vi "test MSS.vi"() -> ()   [LabVIEW 2023]
uses:
  Measure and Stimulus Subsystems/Measure and Stimulus Subsystems.lvclass
  Virtual Instrs/Virt Red-y Read Write/Virt Red-y Read Write.lvclass
  Configurations/Pressure Control CFG/Red-y Pressure Control CFG.lvclass
  Configurations/Pressure Control CFG Simulated/Red-y Pressure Control CFG Simulated.lvclass
panel:
  out "Pressure Scaling Max":variant
  out "Signal Type AI":variant
  out "Pressure":variant
  out "Output":variant
  out "Temperature":variant
  out "Flow":variant
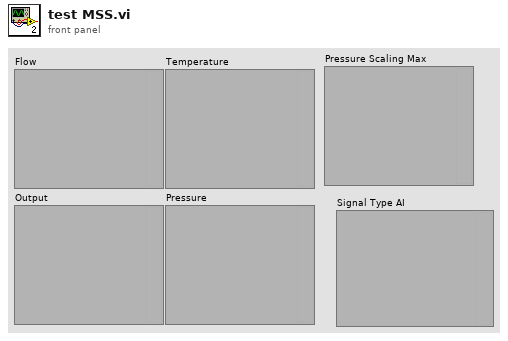
[diagram p1: front panel]
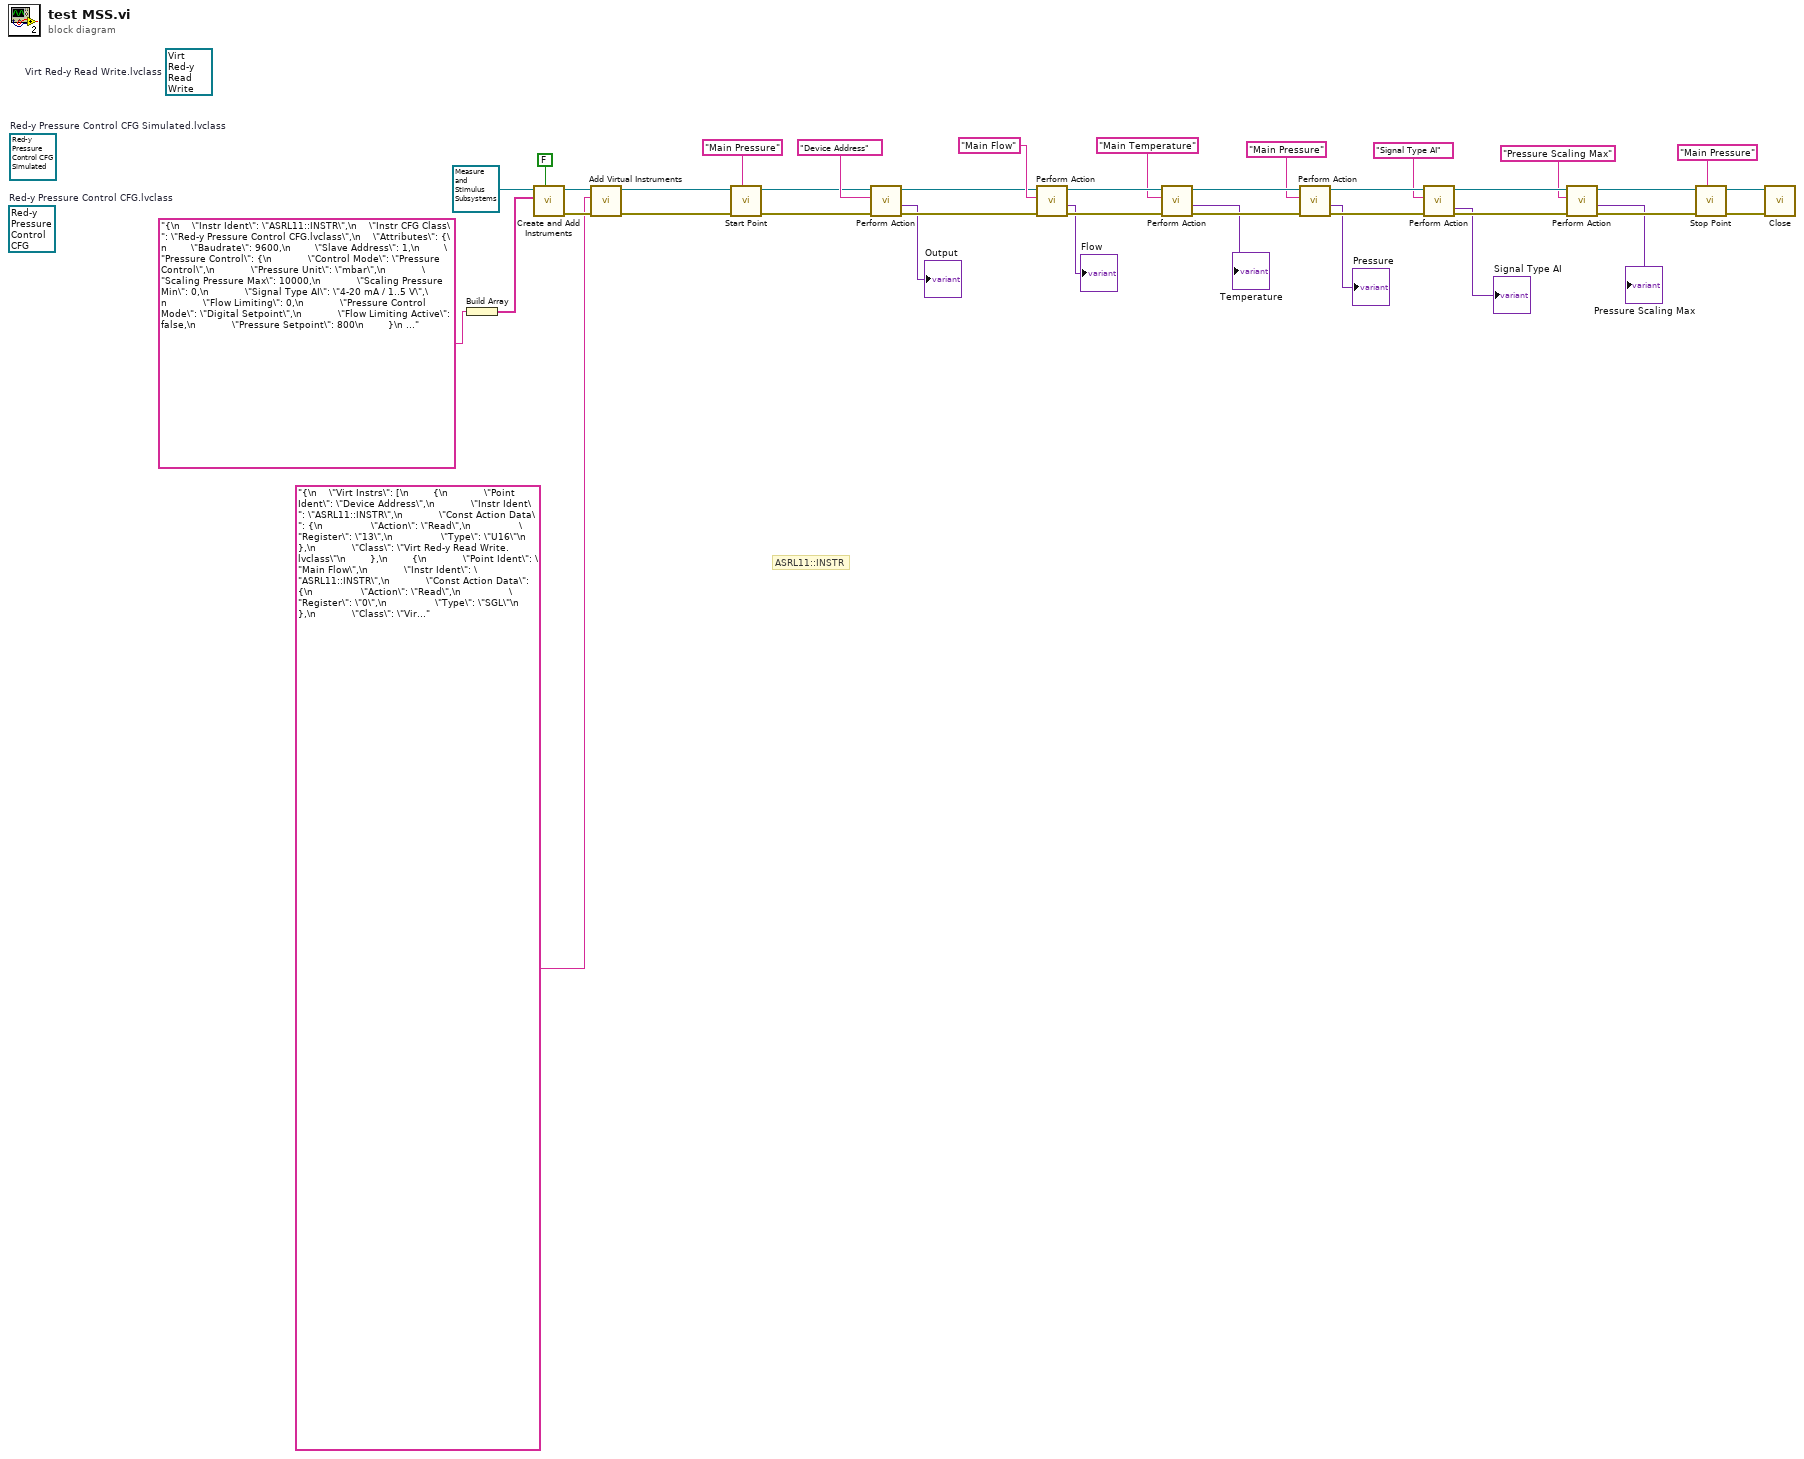
[diagram p0: block diagram]
diagram:
  (unwired) refnum<class "Red-y Pressure Control CFG Simulated.lvclass"> refnum  # Red-y Pressure Control CFG Simulated.lvclass
  (unwired) refnum<class "Red-y Pressure Control CFG.lvclass"> refnum  # Red-y Pressure Control CFG.lvclass
  (unwired) refnum<class "Virt Red-y Read Write.lvclass"> refnum  # Virt Red-y Read Write.lvclass
  # "ASRL11::INSTR"
  n1 = Build Array("{\n    \"Instr Ident\": \"ASRL11::INSTR\",\n    \"Instr CFG Class\": \"Red-y Pressure Control CFG.lvclass\",\n    \"Attributes\": {\n        \"Baudrate\": 9600,\n        \"Slave Address\": 1,\n        \"Pressure Control\": {\n            \"Control Mode\": \"Pressure Control\",\n            \"Pressure Unit\": \"mbar\",\n            \"Scaling Pressure Max\": 10000,\n            \"Scaling Pressure Min\": 0,\n            \"Signal Type AI\": \"4-20 mA / 1..5 V\",\n            \"Flow Limiting\": 0,\n            \"Pressure Control Mode\": \"Digital Setpoint\",\n            \"Flow Limiting Active\": false,\n            \"Pressure Setpoint\": 800\n        }\n    }\n}") -> (w35:string[])
  n2 = call "Create and Add Instruments.vi"("Is Target?"=FALSE, "Physical Intr CFGs"=w35, "MSS in"=refnum<class "Measure and Stimulus Subsystems.lvclass"> refnum ("HAL GOOP4.lvlib:Measure and Stimulus Subsystems.lvclass")) -> ("Error Out"=w38:errorcluster, "MSS out"=w37:refnum<class "Measure and Stimulus Subsystems.lvclass">)  [unwired: 6 in, 1 out]
  n3 = call "Add Virtual Instruments.vi"("error in"=w38, "<JSON CFG>"="{\n    \"Virt Instrs\": [\n        {\n            \"Point Ident\": \"Device Address\",\n            \"Instr Ident\": \"ASRL11::INSTR\",\n            \"Const Action Data\": {\n                \"Action\": \"Read\",\n                \"Register\": \"13\",\n                \"Type\": \"U16\"\n            },\n            \"Class\": \"Virt Red-y Read Write.lvclass\"\n        },\n        {\n            \"Point Ident\": \"Main Flow\",\n            \"Instr Ident\": \"ASRL11::INSTR\",\n            \"Const Action Data\": {\n                \"Action\": \"Read\",\n                \"Register\": \"0\",\n                \"Type\": \"SGL\"\n            },\n            \"Class\": \"Virt Red-y Read Write.lvclass\"\n        },\n        {\n            \"Point Ident\": \"Main Temperature\",\n            \"Instr Ident\": \"ASRL11::INSTR\",\n            \"Const Action Data\": {\n                \"Action\": \"Read\",\n                \"Register\": \"2\",\n                \"Type\": \"SGL\"\n            },\n            \"Class\": \"Virt Red-y Read Write.lvclass\"\n        },\n        {\n            \"Point Ident\": \"Main Pressure\",\n            \"Instr Ident\": \"ASRL11::INSTR\",\n            \"Const Action Data\": {\n                \"Action\": \"Read\",\n                \"Register\": \"5F00\",\n                \"Type\": \"SGL\"\n            },\n            \"Class\": \"Virt Red-y Read Write.lvclass\"\n        },\n        {\n            \"Point Ident\": \"Main Pressure Setpoint\",\n            \"Instr Ident\": \"ASRL11::INSTR\",\n            \"Const Action Data\": {\n                \"Action\": \"Write\",\n                \"Register\": \"5F06\",\n                \"Type\": \"SGL\"\n            },\n            \"Class\": \"Virt Red-y Read Write.lvclass\"\n        },\n        {\n            \"Point Ident\": \"Signal Type AI\",\n            \"Instr Ident\": \"ASRL11::INSTR\",\n            \"Const Action Data\": {\n                \"Action\": \"Read\",\n                \"Register\": \"4085\",\n                \"Type\": \"U16\"\n            },\n            \"Class\": \"Virt Red-y Read Write.lvclass\"\n        },\n\t\t        {\n            \"Point Ident\": \"Pressure Scaling Max\",\n            \"Instr Ident\": \"ASRL11::INSTR\",\n            \"Const Action Data\": {\n                \"Action\": \"Read\",\n                \"Register\": \"5F04\",\n                \"Type\": \"SGL\"\n            },\n            \"Class\": \"Virt Red-y Read Write.lvclass\"\n        }\n    ]\n}", "MSS in"=w37) -> ("error out"=w33:errorcluster, "MSS out"=w17:refnum<class "Measure and Stimulus Subsystems.lvclass">)  [unwired: 6 in, 1 out]
  n4 = call "Start Point.vi"("Task-Point Ident"="Main Pressure", "error in"=w33, "MSS in"=w17) -> ("error out"=w18:errorcluster, "MSS out"=w16:refnum<class "Measure and Stimulus Subsystems.lvclass">)  [unwired: 7 in]
  n5 = call "Perform Action.vi"("error in"=w18, "Point Ident"="Device Address", "MSS in"=w16) -> ("error out"=w25:errorcluster, "Output"=→"Output":variant, "MSS out"=w24:refnum<class "Measure and Stimulus Subsystems.lvclass">)  [unwired: 5 in, 1 out]
  n6 = call "Perform Action.vi"("error in"=w25, "Point Ident"="Main Flow" ("Task-Point Idents"), "MSS in"=w24) -> ("error out"=w32:errorcluster, "Output"=→"Flow":variant, "MSS out"=w28:refnum<class "Measure and Stimulus Subsystems.lvclass">)  [unwired: 5 in, 1 out]
  n7 = call "Perform Action.vi"("error in"=w32, "Point Ident"="Main Temperature", "MSS in"=w28) -> ("error out"=w29:errorcluster, "Output"=→"Temperature":variant, "MSS out"=w20:refnum<class "Measure and Stimulus Subsystems.lvclass">)  [unwired: 5 in, 1 out]
  n8 = call "Perform Action.vi"("error in"=w29, "Point Ident"="Main Pressure", "MSS in"=w20) -> ("error out"=w21:errorcluster, "Output"=→"Pressure":variant, "MSS out"=w9:refnum<class "Measure and Stimulus Subsystems.lvclass">)  [unwired: 5 in, 1 out]
  n9 = call "Perform Action.vi"("error in"=w21, "Point Ident"="Signal Type AI", "MSS in"=w9) -> ("error out"=w10:errorcluster, "Output"=→"Signal Type AI":variant, "MSS out"=w5:refnum<class "Measure and Stimulus Subsystems.lvclass">)  [unwired: 5 in, 1 out]
  n10 = call "Perform Action.vi"("error in"=w10, "Point Ident"="Pressure Scaling Max", "MSS in"=w5) -> ("error out"=w6:errorcluster, "Output"=→"Pressure Scaling Max":variant, "MSS out"=w4:refnum<class "Measure and Stimulus Subsystems.lvclass">)  [unwired: 5 in, 1 out]
  n11 = call "Stop Point.vi"("Task-Point Idents"="Main Pressure", "error in"=w6, "MSS in"=w4) -> ("error out"=w14:errorcluster, "MSS out"=w13:refnum<class "Measure and Stimulus Subsystems.lvclass">)  [unwired: 7 in]
  n12 = call "Close.vi"("error in"=w14, "MSS in"=w13) -> ()  [unwired: 8 in, 2 out]
